vi "Spaneingang manipulieren.vi"(7 "Analysator Auswahl":T2 {"Analysator Auswahl 12" items=["----"=100, "FT-IR"=0, "TEST"=1]; "Analysator Auswahl 11" items=["----"=100, "FT-IR"=0, "TEST"=1]; "Analysator Auswahl 10" items=["----"=100, "FT-IR"=0, "TEST"=1]; "Analysator Auswahl 9" items=["----"=100, "FT-IR"=0, "TEST"=1]; "Analysator Auswahl 8" items=["----"=100, "FT-IR"=0, "TEST"=1]; "Analysator Auswahl 7" items=["----"=100, "FT-IR"=0, "TEST"=1]; "Analysator Auswahl 6" items=["----"=100, "FT-IR"=0, "TEST"=1]; "Analysator Auswahl 5" items=["----"=100, "FT-IR"=0, "TEST"=1]; "Analysator Auswahl 4" items=["----"=100, "FT-IR"=0, "TEST"=1]; "Analysator Auswahl 3" items=["----"=100, "FT-IR"=0, "TEST"=1]; "Analysator Auswahl 2" items=["----"=100, "FT-IR"=0, "TEST"=1]; "Analysator Auswahl" items=["----"=100, "FT-IR"=0, "PMA"=1]}, 8 "error in (no error)":errorcluster caption="Fehler (Eingang, kein Fehler)", 10 "Betriebsdaten":T1[](array[typedef])) -> (0 "error out":errorcluster caption="Fehler (Ausgang)", 2 "Betriebsdaten":T1[](array[typedef]))   [LabVIEW 2020, in "Analysator Definition.lvlib"]
uses:
  Seiten/CalGas Aufschaltung/Cluster Auswahl Analysator.ctl
  Seiten/CalGas Aufschaltung/Analysator Auswahl.ctl
  Betriebsdaten Komponente.ctl
  Analysator Definition.lvlib
  Seiten/CalGas Aufschaltung/CalGas Aufschaltung.lvlib
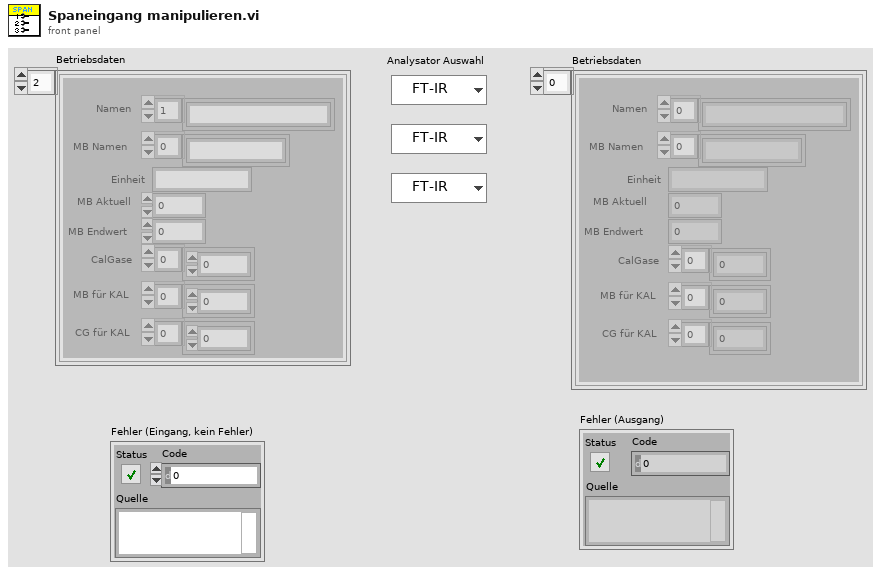
[diagram p1: front panel]
types:
  T1 = typedef "Analysator Definition.lvlib/Betriebsdaten Komponente.ctl" = cluster{"Namen":string[], "MB Namen":string[], "Einheit":string, "MB Aktuell":u16, "MB Endwert":u16, "CalGase":u16[], "MB für KAL":u16[], "CG für KAL":u16[]}
  T2 = typedef "CalGas Aufschaltung.lvlib/Cluster Auswahl Analysator.ctl" = cluster{"Analysator Auswahl":T3, "Analysator Auswahl 2":T3, "Analysator Auswahl 3":T3, "Analysator Auswahl 4":T3, "Analysator Auswahl 5":T3, "Analysator Auswahl 6":T3, "Analysator Auswahl 7":T3, "Analysator Auswahl 8":T3, "Analysator Auswahl 9":T3, "Analysator Auswahl 10":T3, "Analysator Auswahl 11":T3, "Analysator Auswahl 12":T3}
  T3 = typedef "CalGas Aufschaltung.lvlib/Analysator Auswahl.ctl" = u16
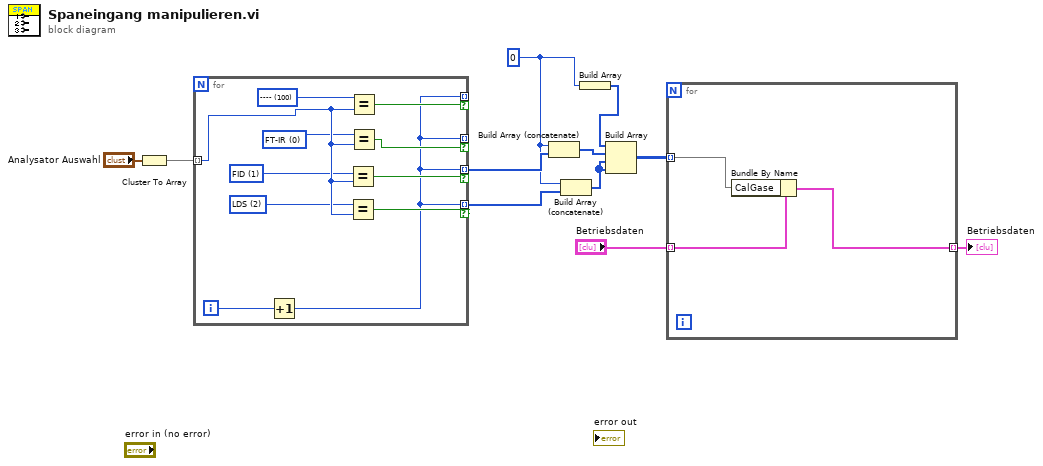
[diagram p0: block diagram]
diagram:
  w1 = 0
  n1 = Cluster To Array(cluster="Analysator Auswahl") -> (array=w10:T3[])
  n2 = for {
    tunnel: w10 -> [w22] mode=indexing
    tunnel: [w12] -> _ mode=indexing if=w17
    tunnel: [w12] -> _ mode=indexing if=w16
    tunnel: [w12] -> w8 mode=indexing if=w15
    tunnel: [w12] -> w7 mode=indexing if=w13
    i -> [w14]
    w18 = T3 2 items=["----"=100, "FT-IR"=0, "FID"=1, "LDS"=2] ("Analysator Auswahl")
    w19 = T3 1 items=["----"=100, "FT-IR"=0, "FID"=1, "LDS"=2] ("Analysator Auswahl")
    w20 = T3 0 items=["----"=100, "FT-IR"=0, "FID"=1, "LDS"=2] ("Analysator Auswahl")
    w21 = T3 100 items=["----"=100, "FT-IR"=0, "FID"=1, "LDS"=2] ("Analysator Auswahl")
    n3 = Increment(x=w14) -> (x+1=w12:i32)
    n4 = Equal?(x=w19, y=w22) -> (x = y?=w15:bool)
    n5 = Equal?(x=w18, y=w22) -> (x = y?=w13:bool)
    n6 = Equal?(x=w21, y=w22) -> (x = y?=w17:bool)
    n7 = Equal?(x=w20, y=w22) -> (x = y?=w16:bool)
  }
  n8 = Build Array (concatenate)(w1, w8) -> (w3:i32[])
  n9 = Build Array (concatenate)(w1, w7) -> (w2:i32[])
  n10 = Build Array(w1) -> (w5:i32[])
  n11 = Build Array(w5, w3, w2, w2) -> (w6:i32[][])
  n12 = for {
    tunnel: "Betriebsdaten" -> [w25] mode=indexing
    tunnel: [w24] -> w4 mode=indexing
    tunnel: w6 -> [w23] mode=indexing
    n13 = Bundle By Name(cluster=w25, "CalGase"=w23) -> (w24:T1)
  }
  "Betriebsdaten" <- w4
